vi "Program07.vi"() -> ()   [LabVIEW 2020]
panel:
  in  "stop":bool
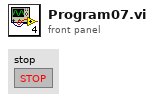
[diagram p1: front panel]
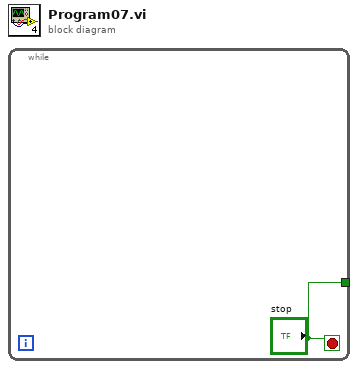
[diagram p0: block diagram]
diagram:
  n1 = while {
    tunnel: ["stop"] -> _
    stop <- "stop" stop-if-true
  }
